vi "Replace GUIDs in Constants VI.vi"(8 "error in":errorcluster, 10 "guid map":map{string, string}(c390), 11 "VI in":refnum<vi>) -> (0 "error out":errorcluster, 3 "VI out":refnum<vi>)   [LabVIEW 2020, in "GUID Tool.lvlib"]
uses:
  GUID Tool.lvlib
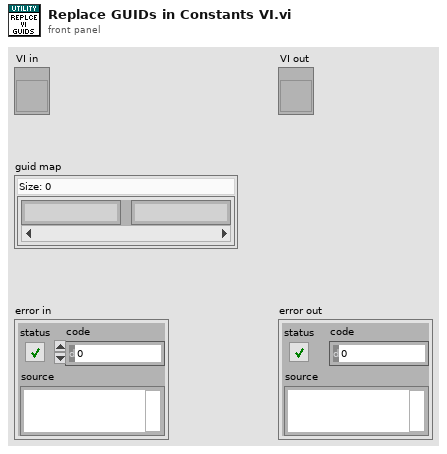
[diagram p1: front panel]
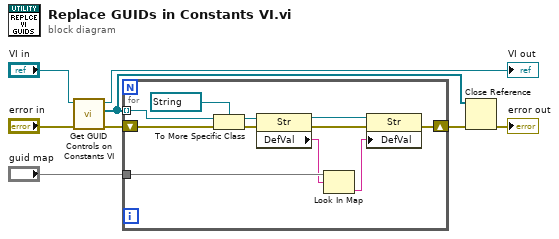
[diagram p0: block diagram]
diagram:
  n1 = call "Get GUID Controls on Constants VI.vi"("error in"="error in", "VI in"="VI in") -> ("error out"=w3:errorcluster, "GUID controls"=w1:refnum<vi>[], "VI out"=→"VI out":refnum<vi>)  [unwired: 7 in]
  n2 = for {
    tunnel: w1 -> [w19] mode=indexing
    shift-right: [w9] -> w5
    shift-left: w3 -> [w15]
    tunnel: "guid map" -> [w14]
    n3 = To More Specific Class(target class=refnum<vi> refnum ("GUID.Import Frames"), reference=w19, error in=w15) -> (specific class reference=w17:refnum<vi>, error out=w16:errorcluster)
    n4 = property class="Str"(reference=w17, error in=w16) -> (reference out=w11:refnum<vi>, error out=w12:errorcluster, "DefVal"=w13:string)
    n5 = Look In Map(map=w14, key=w13) -> (value=w10:string)  [unwired: 1 in, 1 out]
    n6 = property class="Str"(reference=w11, error in=w12, "DefVal"=w10) -> (error out=w9:errorcluster)  [unwired: 1 out]
  }
  n7 = Close Reference(reference=w1, error in (no error)=w5) -> (error out=→"error out":errorcluster)
